vi "XML pose.vi"(8 "tag":string, 11 "String":string) -> (0 "Pose":dbl[][](array[numeric]), 2 "T":T1=[[0.016284994521607307, 0.9998576764567041, 0.0044074691186384496, -12.095922523672678], [0.9998670931969393, -0.01628143110047913, -0.0008431744914288715, -1019.3924117975101], [-0.0007712945830650122, 0.004420614427981981, -0.999989931585686, 240.25900755427352], [0.0, 0.0, 0.0, 1.0]] format="%.3f", 3 "Object":string)   [LabVIEW 2013]
uses:
  <vilib>/Analysis/Matrix/Datatypes/RealMatrix.ctl
  <vilib>/Analysis/Matrix/NI_Matrix.lvlib
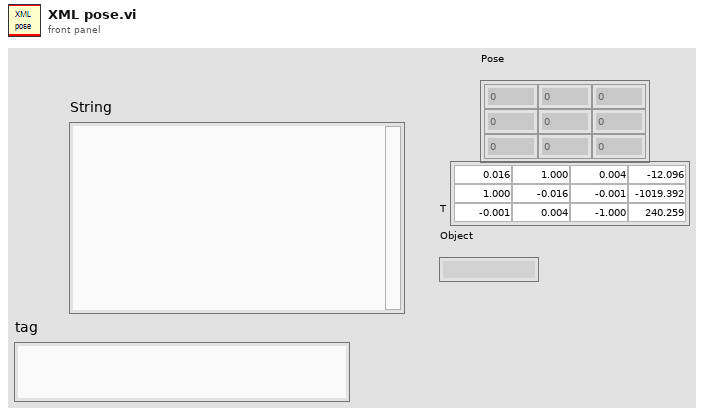
[diagram p1: front panel]
types:
  T1 = typedef "NI_Matrix.lvlib/RealMatrix.ctl" = dbl[][]
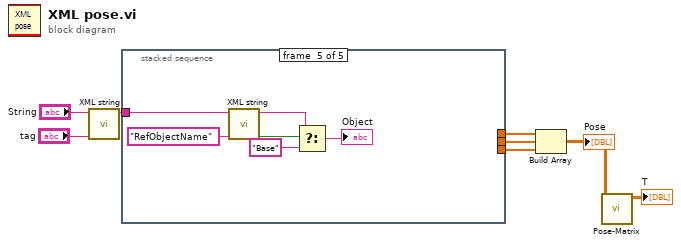
[diagram p0: block diagram]
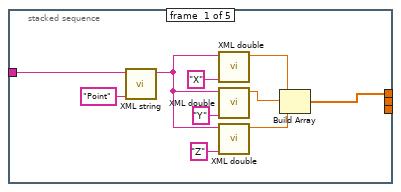
[diagram p2: hidden frame]
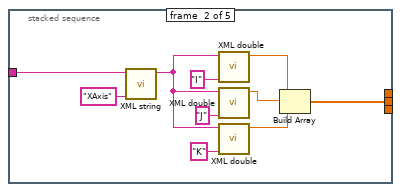
[diagram p3: hidden frame]
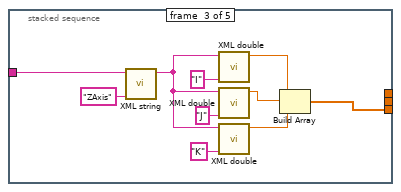
[diagram p4: hidden frame]
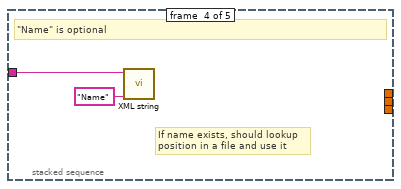
[diagram p5: hidden frame]
diagram:
  n1 = call "XML string.vi"("tag"="tag", "String"="String") -> ("string"=w6:string)  [unwired: 8 in, 1 out]
  n2 = stacked-sequence {
    tunnel: w6 -> [w17 w27 w37 w40 w46]
    tunnel: [_ _ w29 _ _] -> w3
    tunnel: [_ w19 _ _ _] -> w4
    tunnel: [w9 _ _ _ _] -> w5
    frame #0 {
      n3 = call "XML string.vi"("tag"="Point", "String"=w17) -> ("string"=w16:string)  [unwired: 8 in, 1 out]
      n4 = call "XML double.vi"("tag"="X", "String"=w16) -> ("int"=w11:dbl)  [unwired: 9 in]
      n5 = call "XML double.vi"("tag"="Y", "String"=w16) -> ("int"=w12:dbl)  [unwired: 9 in]
      n6 = call "XML double.vi"("tag"="Z", "String"=w16) -> ("int"=w10:dbl)  [unwired: 9 in]
      n7 = Build Array(w11, w12, w10) -> (w9:dbl[])
    }
    frame #1 {
      n8 = call "XML string.vi"("tag"="XAxis", "String"=w27) -> ("string"=w26:string)  [unwired: 8 in, 1 out]
      n9 = call "XML double.vi"("tag"="I", "String"=w26) -> ("int"=w21:dbl)  [unwired: 9 in]
      n10 = call "XML double.vi"("tag"="J", "String"=w26) -> ("int"=w22:dbl)  [unwired: 9 in]
      n11 = call "XML double.vi"("tag"="K", "String"=w26) -> ("int"=w20:dbl)  [unwired: 9 in]
      n12 = Build Array(w21, w22, w20) -> (w19:dbl[])
    }
    frame #2 {
      n13 = call "XML string.vi"("tag"="ZAxis", "String"=w37) -> ("string"=w36:string)  [unwired: 8 in, 1 out]
      n14 = call "XML double.vi"("tag"="I", "String"=w36) -> ("int"=w31:dbl)  [unwired: 9 in]
      n15 = call "XML double.vi"("tag"="J", "String"=w36) -> ("int"=w32:dbl)  [unwired: 9 in]
      n16 = call "XML double.vi"("tag"="K", "String"=w36) -> ("int"=w30:dbl)  [unwired: 9 in]
      n17 = Build Array(w31, w32, w30) -> (w29:dbl[])
    }
    frame #3 {
      # "If name exists, should lookup\nposition in a file and use it"
      # "\"Name\" is optional"
      n18 = call "XML string.vi"("tag"="Name", "String"=w40) -> ()  [unwired: 8 in, 2 out]
    }
    frame #4 {
      n19 = call "XML string.vi"("tag"="RefObjectName", "String"=w46) -> ("Tag Found"=w44:bool, "string"=w43:string)  [unwired: 8 in]
      n20 = Select(t=w43, s=w44, f="Base") -> (s? t:f=→"Object":string)
    }
  }
  n21 = Build Array(w5, w4, w3) -> (w2:dbl[][])
  "Pose" <- w2
  n22 = call "Pose-Matrix.vi"("pose"=w2) -> ("T"=→"T":T1)  [unwired: 9 in, 1 out]
